vi "evo irimager to palette save png.vi"(5 "palette_scale":i32, 6 "palette":i32, 7 "path":string, 9 "h":i32, 10 "w":i32, 11 "thermal_data":u16[](array[numeric])) -> (2 "function return":i32, 3 "thermal_data out":u16[](array[numeric]))   [LabVIEW 2024, in "libirimager_direct_binding.lvlib"]
doc: "DIRECT_API int evo_irimager_to_palette_save_png(unsigned short* thermal_data, int w, int h, const char* path, int palette, int palette_scale);"
uses:
  libirimager_direct_binding.lvlib
  libirimager.dll
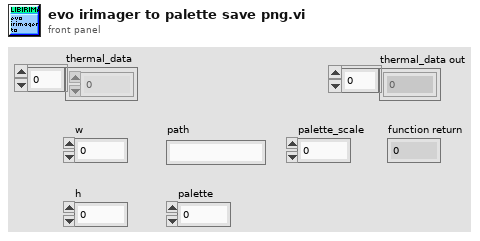
[diagram p1: front panel]
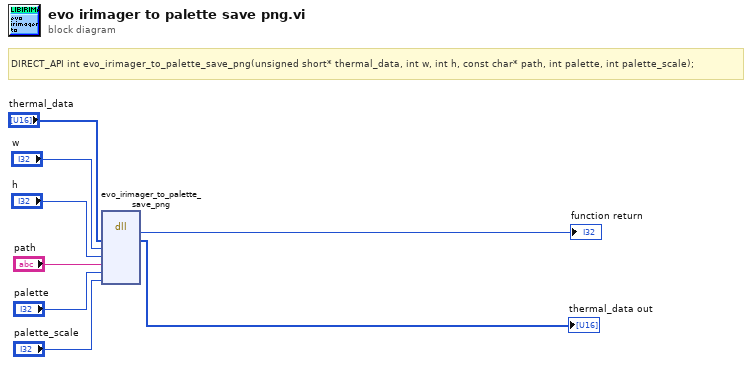
[diagram p0: block diagram]
diagram:
  # "DIRECT_API int evo_irimager_to_palette_save_png(unsigned short* thermal_data, int w, int h, const char* path, int palette, int palette_scale);"
  n1 = dll-call lib="C:/Users/mayhe/OneDrive/Documents/irDirectSDK/examples/labview/libirimager.dll" fn="evo_irimager_to_palette_save_png"("thermal_data"="thermal_data", "w"="w", "h"="h", "path"="path", "palette"="palette", "palette_scale"="palette_scale") -> ("Rückgabetyp"=→"function return":i32, "thermal_data"=→"thermal_data out":u16[])  [unwired: 8 in, 2 out]
